vi "数据导入工具-main.vi"() -> ()   [LabVIEW 2016]
uses:
  <vilib>/Utility/sysdir.llb/System Directory Type.ctl
  <vilib>/addons/database/Connection.llb/DB Tools Open Connec (String).vi
  <userlib>/_LVST/sqlite_api/Core/Tables/SQLite_List Tables.vi
  <vilib>/addons/database/NI_Database_API.lvlib
  Access/Access Lib.lvlib
panel:
  in  "SQLite Password":string
  in  "Access Password":string
  in  "Sqlite加密":bool
  in  "Sqlite解密":bool
  out "selected path":path caption="所选路径"
  in  "导入日志":string
  in  "导入SQLite":bool
  in  "ACCESS数据表":bool
  in  "列表框":i32[](listbox)
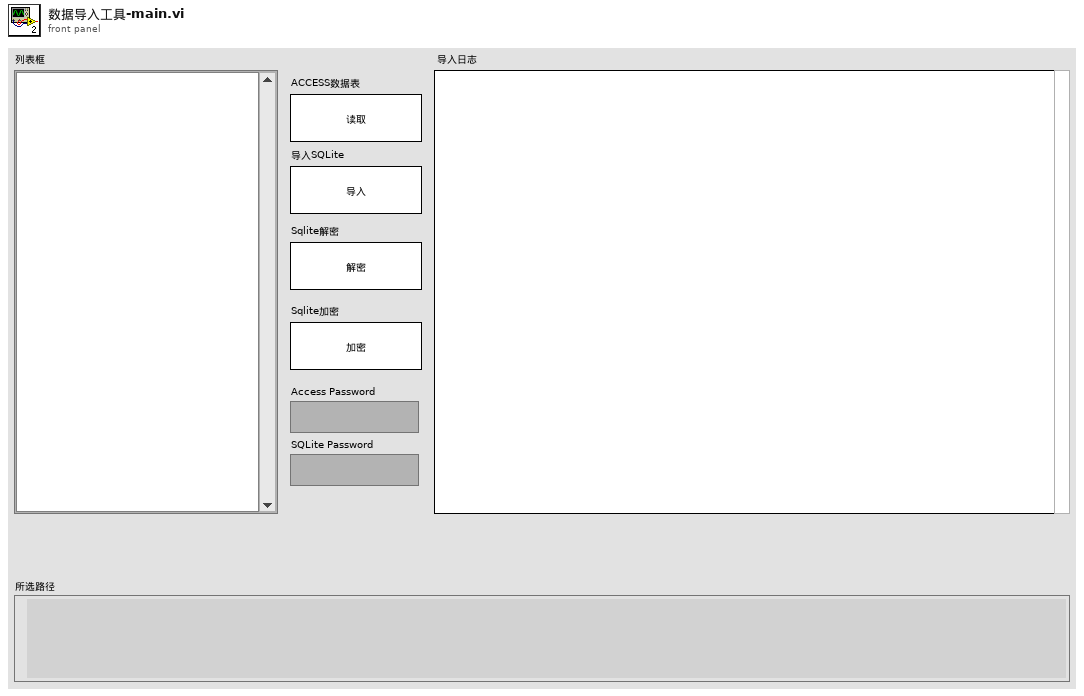
[diagram p1: front panel]
types:
  T1 = typedef "System Directory Type.ctl" = i32
  T2 = typedef "NI_Database_API.lvlib/Conn ObjectReference.ctl" = refnum<k1>
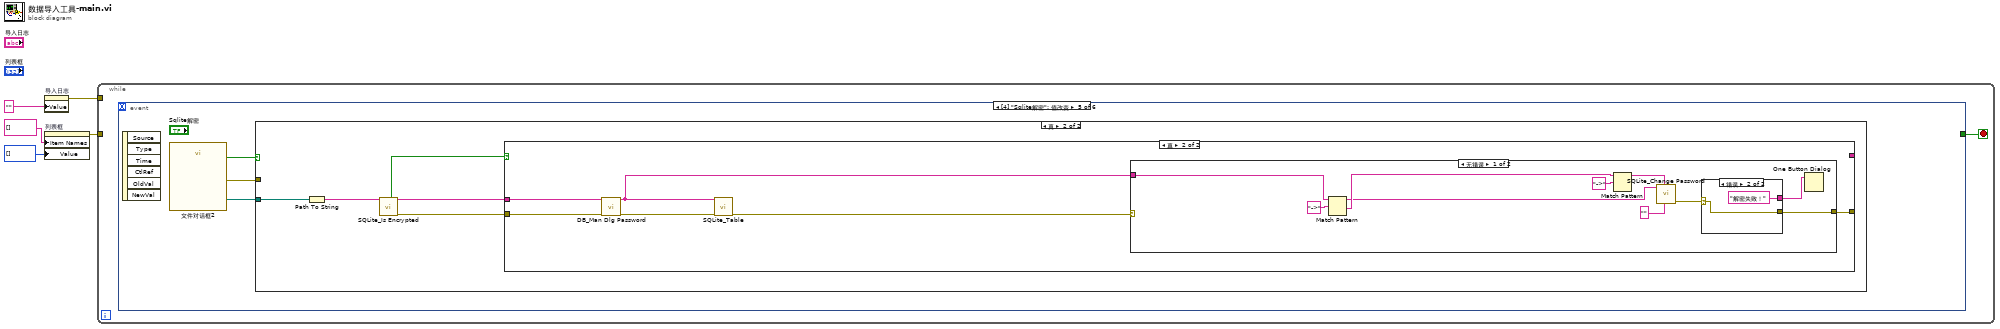
[diagram p0: block diagram]
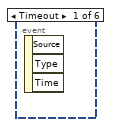
[diagram p2: hidden frame]
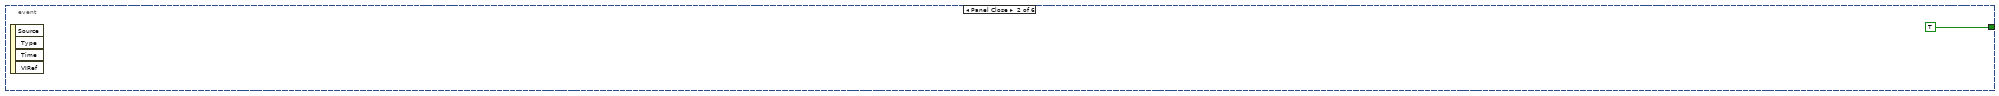
[diagram p3: hidden frame]
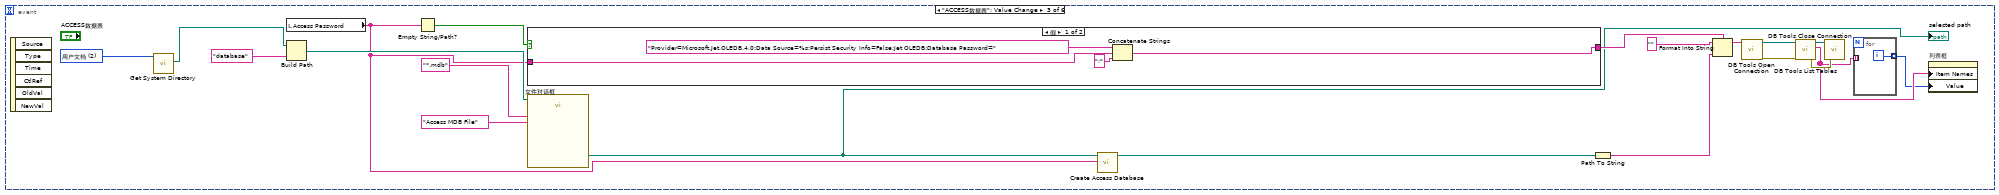
[diagram p4: hidden frame]
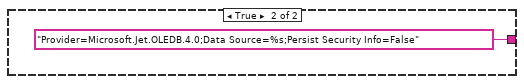
[diagram p5: hidden frame]
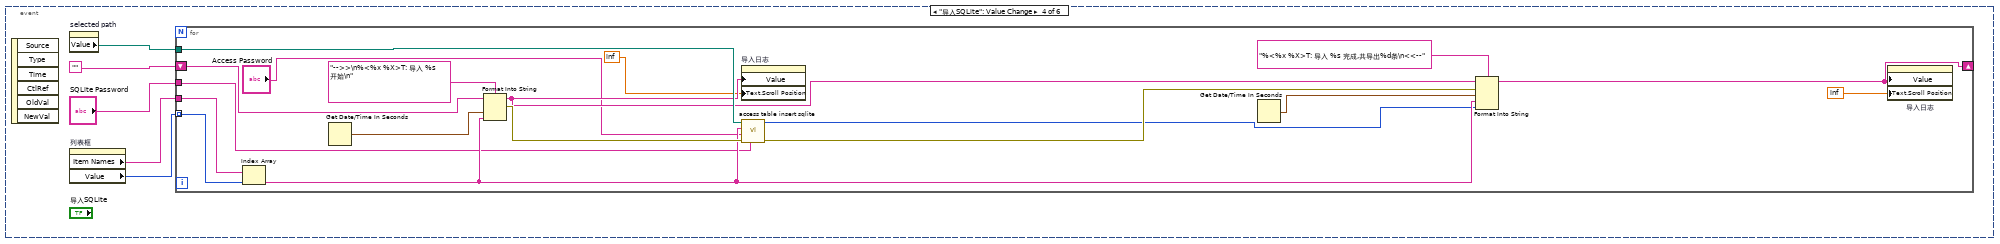
[diagram p6: hidden frame]
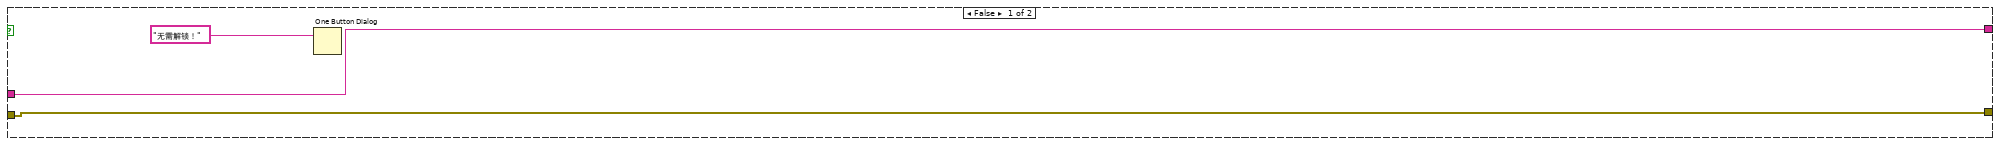
[diagram p8: hidden frame]
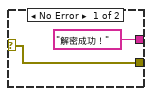
[diagram p9: hidden frame]
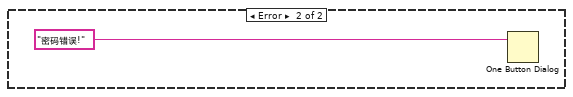
[diagram p10: hidden frame]
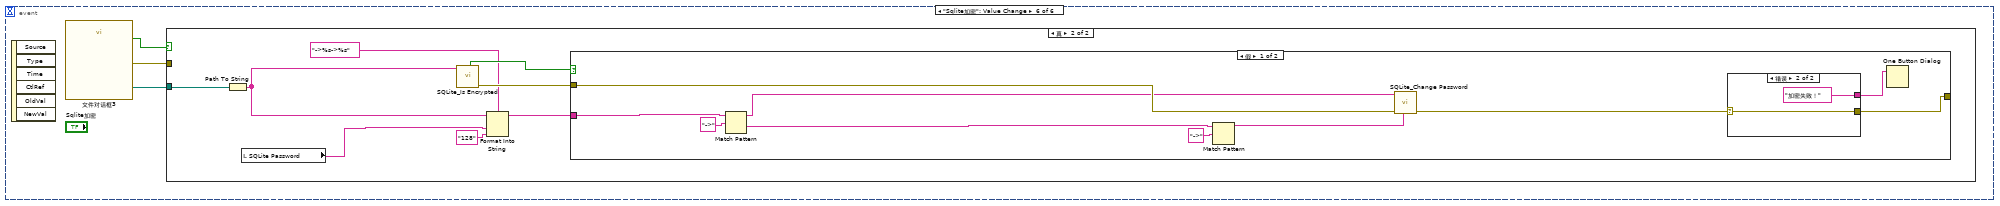
[diagram p11: hidden frame]
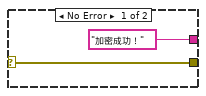
[diagram p13: hidden frame]
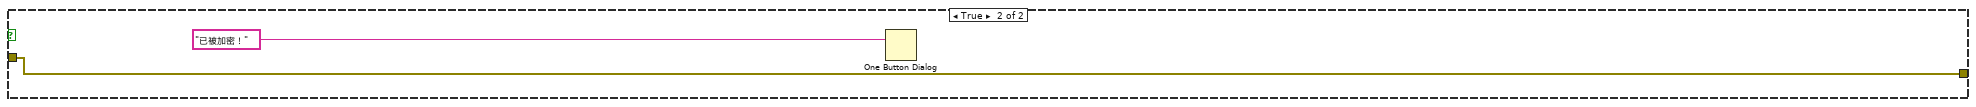
[diagram p14: hidden frame]
diagram:
  n1 = property on="导入日志" class="Str"("Value"="" ("导入日志")) -> (error out=w1:errorcluster)  [unwired: 2 in, 1 out]
  n2 = property on="列表框" class="LstBox (严格)"("Item Names"=string[] [] ("项名"), "Value"=i32[] [] ("列表框")) -> (error out=w3:errorcluster)  [unwired: 2 in, 1 out]
  n3 = while {
    tunnel: w3 -> [_]
    tunnel: w1 -> [_]
    stop <- w6 stop-if-true
    n4 = event shown="[4] \"Sqlite解密\": 值改变" {
      selector: _ -> [_ _ _ _ _ _]
      dyn-events: _ -> [_ _ _ _ _ _]
      timeout: _ -> [_ _ _ _ _ _]
      tunnel: [_ TRUE _ _ _ _] -> w6
      event Timeout {
        n5 = event-data() -> ()  [unwired: 1 in, 3 out]
      }
      event Panel Close {
        n6 = event-data() -> ()  [unwired: 1 in, 4 out]
      }
      event "ACCESS数据表": Value Change {
        w27 = T1 2 items=["用户目录"=0, "用户桌面"=1, "用户文档"=2, "用户应用程序数据"=3, "用户设置"=4, "用户临时目录"=5, "公共文档"=6, "公共应用程序数据"=7, "公共设置"=8, "公共缓存"=13, "系统核心库"=9, "系统安装库"=10, "应用程序文件"=11, "启动盘根目录"=12] ("system directory type")
        n7 = event-data() -> ()  [unwired: 1 in, 6 out]
        n8 = call <vilib>:"Get System Directory.vi"("system directory type"=w27) -> ("system directory"=w26:path)  [unwired: 10 in]
        n9 = local read "Access Password"() -> (w15:string)
        n10 = Build Path(base path=w26, name or relative path="database" ("名称或相对路径")) -> (appended path=w25:path)
        n11 = Empty String/Path?(string/path=w15) -> (empty?=w10:bool)
        n12 = case shown="假" w10 {
          tunnel: [w28 "Provider=Microsoft.Jet.OLEDB.4.0;Data Source=%s;Persist Security Info=False" ("格式字符串")] -> w11
          tunnel: w15 -> [w31 _]
          frame False {
            n13 = Concatenate Strings("Provider=Microsoft.Jet.OLEDB.4.0;Data Source=%s;Persist Security Info=False;Jet OLEDB:Database Password=" ("格式字符串"), w31, ";" ("字符串")) -> (w28:string)
          }
          frame True {
          }
        }
        n14 = call "文件对话框"("start path"=w25, "pattern (all files)"="*.mdb", "pattern label"="Access MDB File") -> ("selected path"=w9:path)  [unwired: 9 in, 3 out]
        "selected path" <- w9
        n15 = call "Create Access Database.vi"("Password"=w15, "路径"=w9) -> ("路径 out"=w14:path)  [unwired: 8 in, 1 out]
        n16 = Path To String(path=w14) -> (string=w13:string)
        n17 = Format Into String(format string=w11, initial string="" ("初始字符串"), w13) -> (resulting string=w8:string)  [unwired: 1 in, 1 out]
        n18 = call-poly <vilib>:"DB Tools Open Connection.vi"("connection information"=w8) -> ("error out"=w21:errorcluster, "connection reference"=w20:T2)  [unwired: 7 in]
        n19 = call <vilib>:"DB Tools List Tables.vi"("error in (no error)"=w21, "connection reference"=w20) -> ("error out"=w18:errorcluster, "tables"=w17:string[], "connection reference out"=w19:T2)  [unwired: 3 in]
        n20 = call <vilib>:"DB Tools Close Connection.vi"("error in (no error)"=w18, "connection reference"=w19) -> ()  [unwired: 5 in, 1 out]
        n21 = for {
          tunnel: w17 -> [_] mode=indexing
          tunnel: [w33] -> w16 mode=indexing
          i -> [w33]
        }
        n22 = property on="列表框" class="LstBox (严格)"("Item Names"=w17, "Value"=w16) -> ()  [unwired: 2 in, 2 out]
      }
      event "导入SQLite": Value Change {
        n23 = event-data() -> ()  [unwired: 1 in, 6 out]
        n24 = property on="selected path" class="Path"() -> ("Value"=w38:path)  [unwired: 2 in, 2 out]
        n25 = property on="列表框" class="LstBox (严格)"() -> ("Item Names"=w36:string[], "Value"=w37:i32[])  [unwired: 2 in, 2 out]
        n26 = for {
          tunnel: w36 -> [w56]
          tunnel: w37 -> [w55] mode=indexing
          tunnel: w38 -> [w54]
          shift-right: [w48] -> _
          shift-left: "" -> [w53]
          tunnel: "SQLite Password" -> [w39]
          n27 = Index Array(array=w56, index=w55) -> (element=w50:string)
          n28 = Get Date/Time In Seconds() -> (seconds since 1Jan1904=w45:timestamp)
          n29 = Format Into String(format string="-->>\n%<%x %X>T: 导入 %s 开始\n" ("格式字符串"), initial string=w53, w45, w50) -> (resulting string=w49:string, error out=w52:errorcluster)  [unwired: 1 in]
          n30 = property on="导入日志" class="Str"("Value"=w49, "Text.Scroll Position"=inf) -> ()  [unwired: 2 in, 2 out]
          n31 = call "access table insert sqlite.vi"("SQLite Password"=w39, "error in (no error)"=w52, "Access Password"="Access Password", "table"=w50, "路径"=w54) -> ("错误输出"=w51:errorcluster, "条数"=w47:i32)  [unwired: 5 in]
          n32 = Get Date/Time In Seconds() -> (seconds since 1Jan1904=w42:timestamp)
          n33 = Format Into String(format string="%<%x %X>T: 导入 %s 完成,共导出%d条\n<<--" ("格式字符串"), initial string=w49, error in=w51, w42, w50, w47) -> (resulting string=w48:string)  [unwired: 1 out]
          n34 = property on="导入日志" class="Str"("Value"=w48, "Text.Scroll Position"=inf) -> ()  [unwired: 2 in, 2 out]
        }
      }
      event "Sqlite解密": Value Change {
        n35 = event-data() -> ()  [unwired: 1 in, 6 out]
        n36 = call "文件对话框2"() -> ("selected path"=w59:path, "exists"=w57:bool, "error out"=w58:errorcluster)  [unwired: 12 in, 1 out]
        n37 = case shown="真" w57 {
          tunnel: w59 -> [_ w64]
          tunnel: w58 -> [_ _]
          frame False {
          }
          frame True {
            n38 = Path To String(path=w64) -> (string=w60:string)
            n39 = call <userlib>:"SQLite_Is Encrypted.vi"("Path"=w60) -> ("error out"=w63:errorcluster, "Path Out"=w62:string, "Encrypted?"=w61:bool)  [unwired: 7 in]
            n40 = case shown="真" w61 {
              tunnel: [w66 w71] -> _
              tunnel: w63 -> [w66 w73]
              tunnel: w62 -> [w67 w72]
              tunnel: [w67 _] -> _
              frame False {
                n41 = One Button Dialog(message="无需解锁！" ("消息")) -> ()  [unwired: 1 in, 1 out]
              }
              frame True {
                n42 = call <userlib>:"DB_Man Dlg Password.vi"("error in (no error)"=w73, "Path in"=w72) -> ("error out"=w69:errorcluster, "Path Out"=w70:string)  [unwired: 8 in]
                n43 = call-poly <userlib>:"SQLite_Table.vi"("DB Path"=w70, "error in (no error)"=w69) -> ("error out"=w68:errorcluster)  [unwired: 6 in, 2 out]
                n44 = case shown="无错误" w68 {
                  tunnel: [w76 _] -> w71
                  tunnel: w70 -> [w75 _]
                  frame No Error {
                    n45 = Match Pattern(string=w75, regular expression="->" ("正则表达式")) -> (before substring=w74:string, after substring=w79:string)  [unwired: 1 in, 2 out]
                    n46 = Match Pattern(string=w79, regular expression="->" ("正则表达式")) -> (before substring=w77:string)  [unwired: 1 in, 3 out]
                    n47 = call <userlib>:"SQLite_Change Password.vi"("New Password (Empty to remove)"="", "Old Password"=w77, "DB Path"=w74) -> ("error out"=w81:errorcluster)  [unwired: 7 in, 1 out]
                    n48 = case shown="错误" w81 {
                      selector: w81 -> [w84 w86]
                      tunnel: ["解密成功！" ("Old Password") "解密失败！" ("Old Password")] -> w83
                      tunnel: [w84 w86] -> w76
                      frame No Error {
                      }
                      frame Error {
                      }
                    }
                    n49 = One Button Dialog(message=w83) -> ()  [unwired: 1 in, 1 out]
                  }
                  frame Error {
                    n50 = One Button Dialog(message="密码错误!" ("消息")) -> ()  [unwired: 1 in, 1 out]
                  }
                }
              }
            }
          }
        }
      }
      event "Sqlite加密": Value Change {
        n51 = event-data() -> ()  [unwired: 1 in, 6 out]
        n52 = call "文件对话框3"() -> ("selected path"=w91:path, "exists"=w89:bool, "error out"=w90:errorcluster)  [unwired: 12 in, 1 out]
        n53 = case shown="真" w89 {
          tunnel: w91 -> [_ w99]
          tunnel: w90 -> [_ _]
          frame False {
          }
          frame True {
            n54 = Path To String(path=w99) -> (string=w94:string)
            n55 = local read "SQLite Password"() -> (w92:string)
            n56 = call <userlib>:"SQLite_Is Encrypted.vi"("Path"=w94) -> ("error out"=w98:errorcluster, "Encrypted?"=w97:bool)  [unwired: 7 in, 1 out]
            n57 = Format Into String(format string="->%s->%s", initial string=w94, w92, "128" ("Enter Password")) -> (resulting string=w93:string)  [unwired: 1 in, 1 out]
            n58 = case shown="假" w97 {
              tunnel: [w109 w115] -> _
              tunnel: w98 -> [w106 w115]
              tunnel: w93 -> [w104 _]
              frame False {
                n59 = Match Pattern(string=w104, regular expression="->" ("正则表达式")) -> (before substring=w103:string, after substring=w101:string)  [unwired: 1 in, 2 out]
                n60 = Match Pattern(string=w101, regular expression="->" ("正则表达式")) -> (before substring=w100:string)  [unwired: 1 in, 3 out]
                n61 = call <userlib>:"SQLite_Change Password.vi"("New Password (Empty to remove)"=w100, "error in (no error)"=w106, "DB Path"=w103) -> ("error out"=w107:errorcluster)  [unwired: 7 in, 1 out]
                n62 = case shown="错误" w107 {
                  selector: w107 -> [w110 w112]
                  tunnel: ["加密成功！" ("Old Password") "加密失败！" ("Old Password")] -> w108
                  tunnel: [w110 w112] -> w109
                  frame No Error {
                  }
                  frame Error {
                  }
                }
                n63 = One Button Dialog(message=w108) -> ()  [unwired: 1 in, 1 out]
              }
              frame True {
                n64 = One Button Dialog(message="已被加密！" ("消息")) -> ()  [unwired: 1 in, 1 out]
              }
            }
          }
        }
      }
    }
  }
